vi "SetInstrumentBase.vi"(0 "object in":refnum<class "Application.lvclass">, 1 "InstrumentBase":refnum<class "InstrumentBase.lvclass">, 5 "error in (no error)":errorcluster) -> (14 "object out":refnum<class "Application.lvclass">, 19 "error out":errorcluster)   [LabVIEW 2019, in "Application.lvclass"]
uses:
  Application.lvclass
  InstrumentBase_class/AD2_SDK_class/InstrumentBase.lvclass
  Application.lvclass/Application.ctl
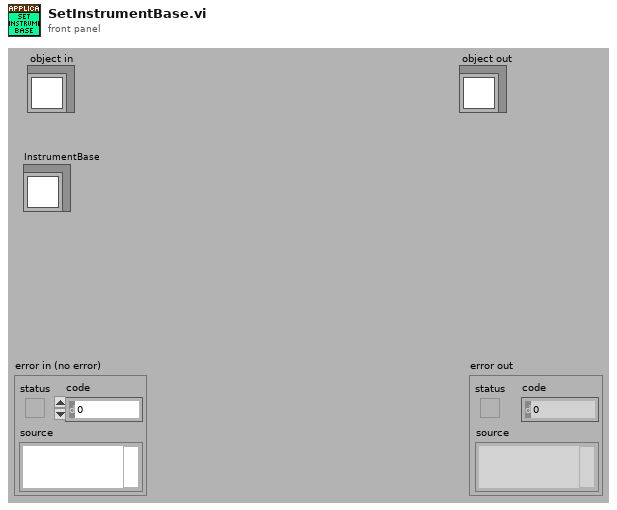
[diagram p1: front panel]
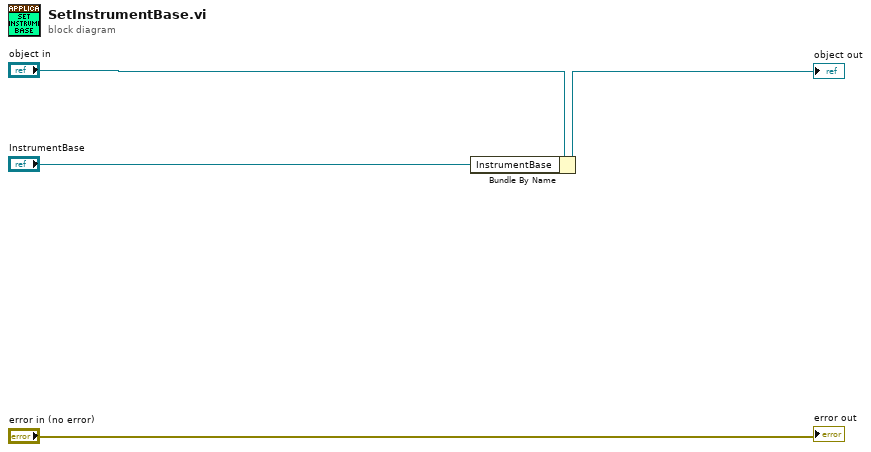
[diagram p0: block diagram]
diagram:
  n1 = Bundle By Name(cluster="object in", "InstrumentBase"="InstrumentBase") -> (→"object out":refnum<class "Application.lvclass">)
  "error out" <- "error in (no error)"
